vi "TrainEditor.vi"(8 "error in (no error)":errorcluster) -> (0 "error out":errorcluster, 1 "Clear Path":bool, 2 "PathData.Path":T1[](array[typedef]))   [LabVIEW 2014]
uses:
  Libraries/Contact Data/Contact.ctl
  Libraries/Contact Data/Position.ctl
  Libraries/Contact Data/Controls.ctl
  Libraries/Contact Data/DestinationCluster.ctl
  Libraries/Contact Data/DesinationControls.ctl
  Libraries/Contact Data/PathData.ctl
  PathFinder/Controls/ShortestPath.ctl
  Libraries/Contact Data/Command.ctl
  Libraries/Contact Data/Contact Data.lvlib
panel:
  in  "Clear Path":bool
  in  "Display Path":bool
  out "PathData":T2
  out "Speed":dbl
  out "SetSpeed":dbl
  out "Contact 2":T3
  in  "Use Copy?":bool
  in  "Destination Template":T6[](array[typedef])
  in  "Name":string
  out "Contact":T3
  in  "Update":i32=1000
  in  "Name display":T8(array[cluster])
  in  "Save ALL Single":bool
  in  "Save for all Dest only":bool
  in  "Destination Array":T6[](array[typedef])
  in  "Delete All":bool
  in  "Delete Index":bool
  in  "Save Destination only":bool
  in  "Load":bool
  out "Contacts":T3[](array[typedef])
  # "ID"
  # "UUID"
  # "Name"
  # "Select"
  # "Destination"
  # "Control"
  # "Timer"
  # "Set Time"
  # "TimeStamp"
  # "Repeat?"
  # "Optional Data"
  # "Distance"
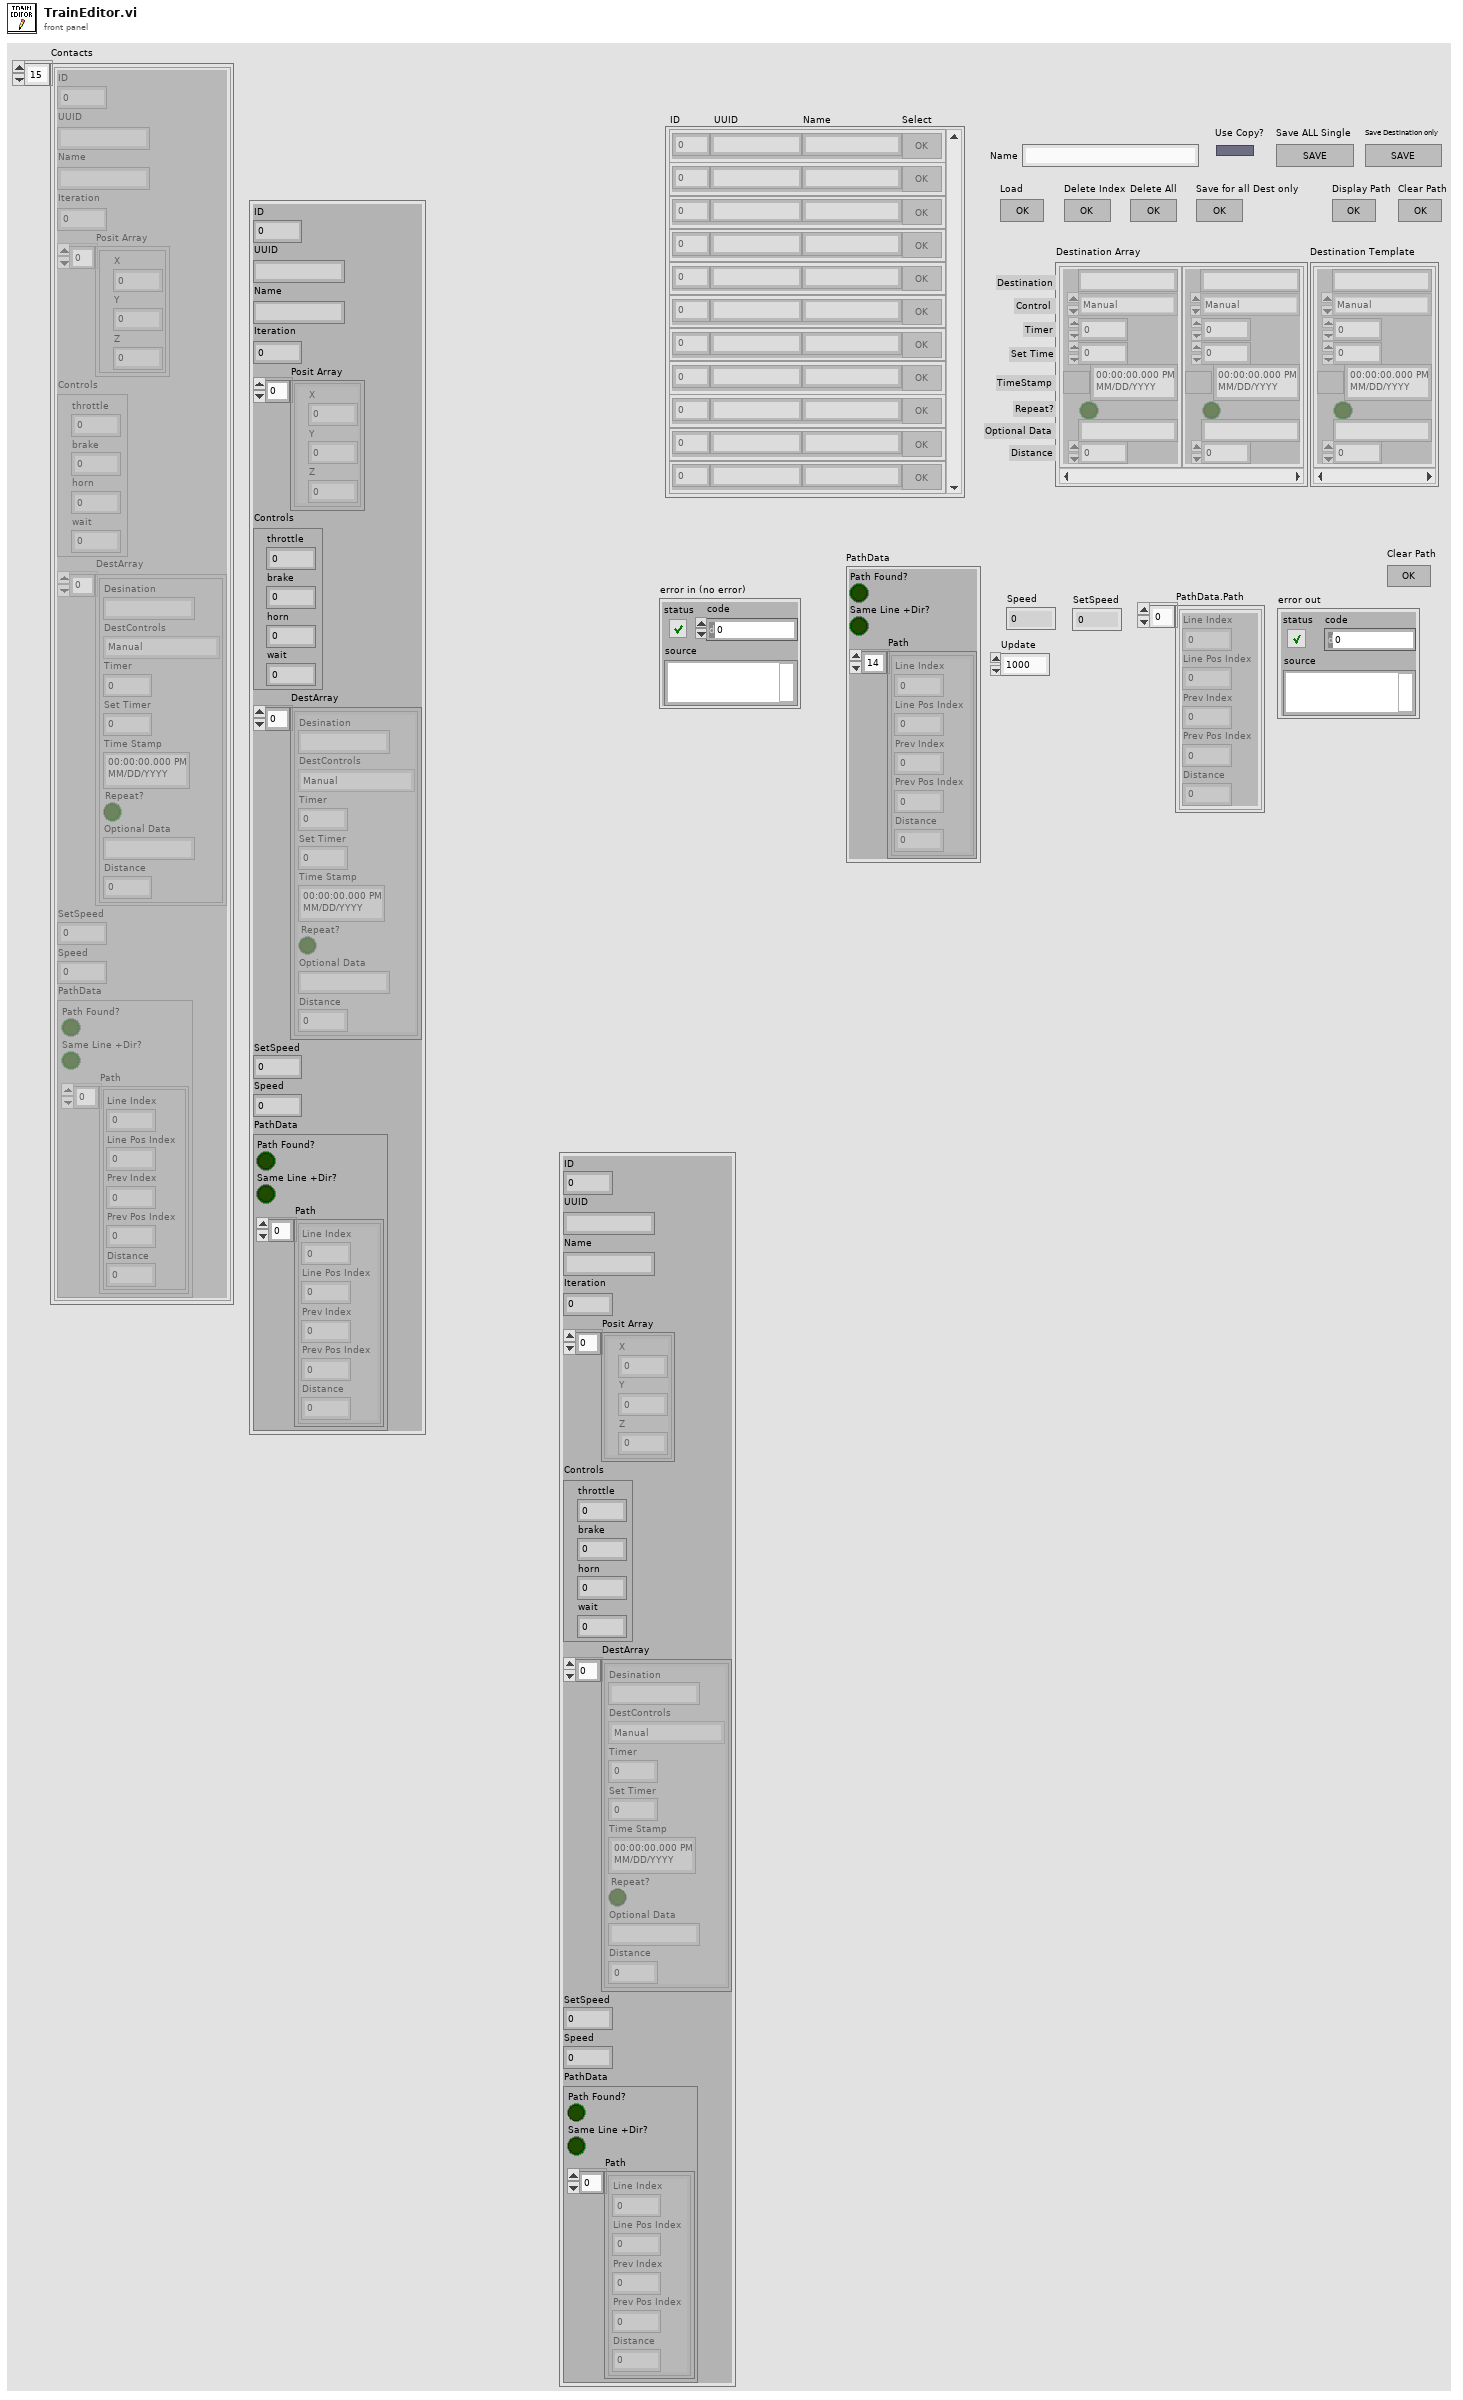
[diagram p1: front panel]
types:
  T1 = typedef "ShortestPath.ctl" = cluster{"Line Index":i32, "Line Pos Index ":i32, "Prev Index ":i32, "Prev Pos Index":i32, "Distance":dbl}
  T2 = typedef "Contact Data.lvlib/PathData.ctl" = cluster{"Path Found?":bool, "Same Line +Dir?":bool, "Path":T1[]}
  T3 = typedef "Contact Data.lvlib/Contact.ctl" = cluster{"ID":u32, "UUID":string, "Name":string, "Iteration":i32, "Posit Array":T4[], "Controls":T5, "DestArray":T6[], "SetSpeed":dbl, "Speed":dbl, "PathData":T2}
  T4 = typedef "Contact Data.lvlib/Position.ctl" = cluster{"X":dbl, "Y":dbl, "Z":dbl}
  T5 = typedef "Contact Data.lvlib/Controls.ctl" = cluster{"throttle":dbl, "brake":dbl, "horn":dbl, "wait":dbl}
  T6 = typedef "Contact Data.lvlib/DestinationCluster.ctl" = cluster{"Desination":string, "DestControls":T7, "Timer":u32, "Set Timer":u32, "Time Stamp":timestamp, "Repeat?":bool, "Optional Data":string, "Distance":dbl}
  T7 = typedef "Contact Data.lvlib/DesinationControls.ctl" = enum16{"Tracker", "Manual", "Stop", "Station DateTime", "Station Timer", "Maintain"}
  T8 = cluster{"ID":u32, "UUID":string, "Name":string, "Select":bool}[]
  T9 = enum32{"Invalid", "Standard", "Closed", "Hidden", "Minimized", "Maximized"}
  T10 = cluster{"ID":u32, "UUID":string, "Name":string, "Select":bool}
  T11 = typedef "Contact Data.lvlib/Command.ctl" = enum16{"Set All Contacts", "Load", "Save", "Get All Data", "Get Single Data (ID)", "Get Single Data", "Set Position", "Set Single Path", "Set Destinations", "Set Controls", "Remove Single Data", "Remove UUID Contact", "Set Single ALL", "Is Data Modified", "Import Data"}
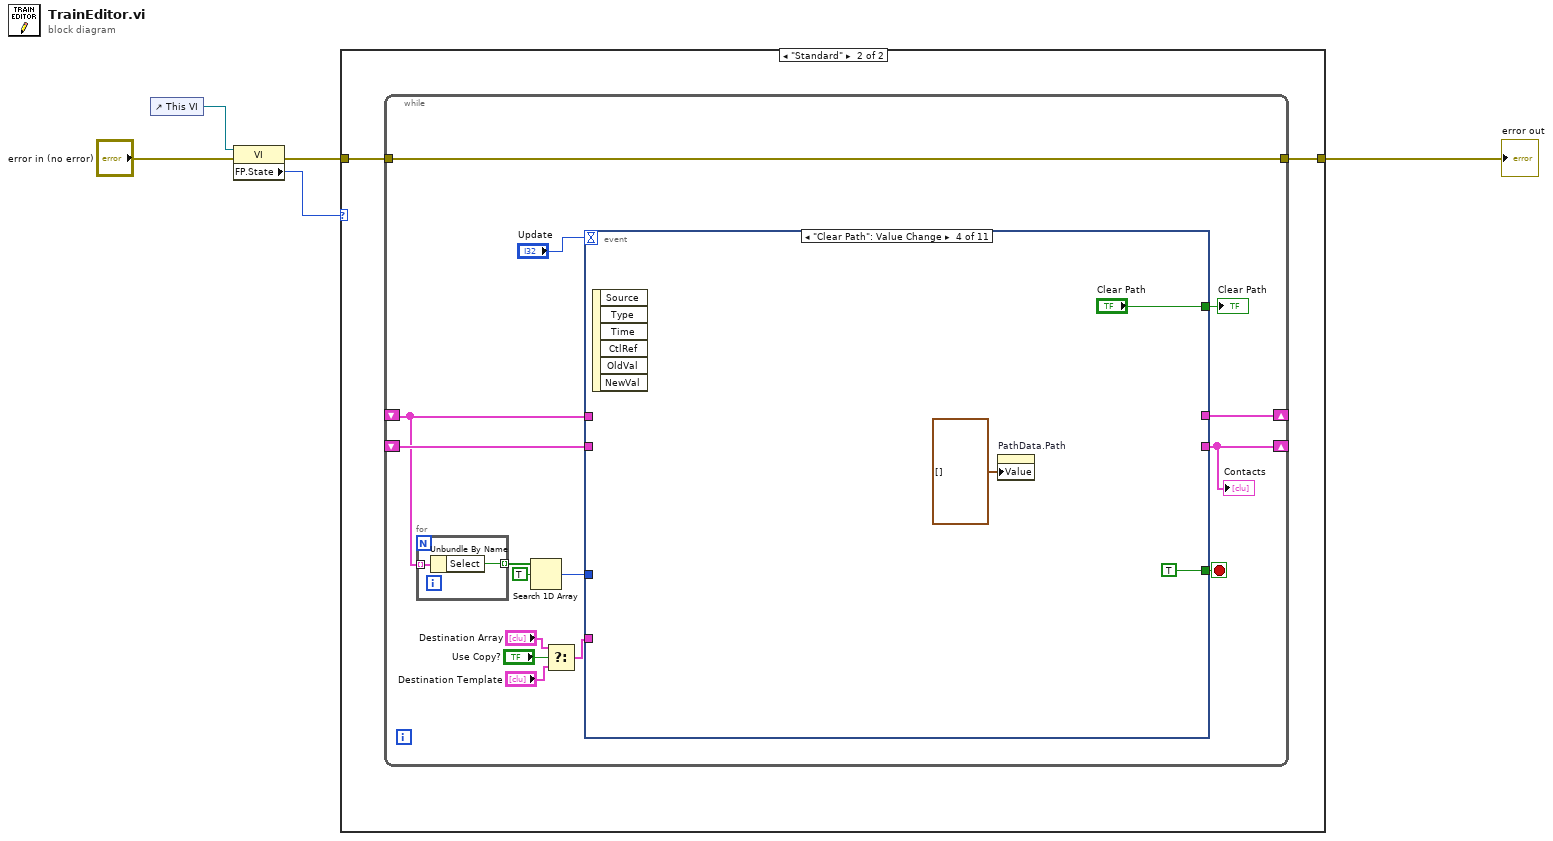
[diagram p0: block diagram]
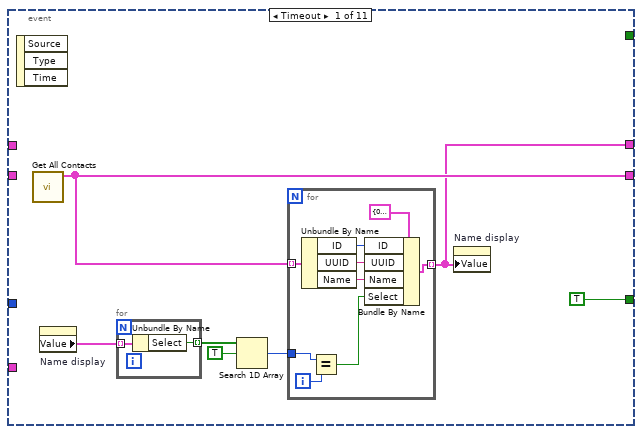
[diagram p3: hidden frame]
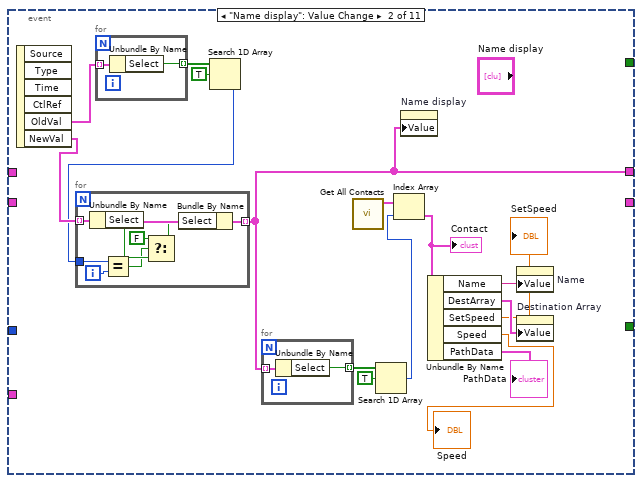
[diagram p4: hidden frame]
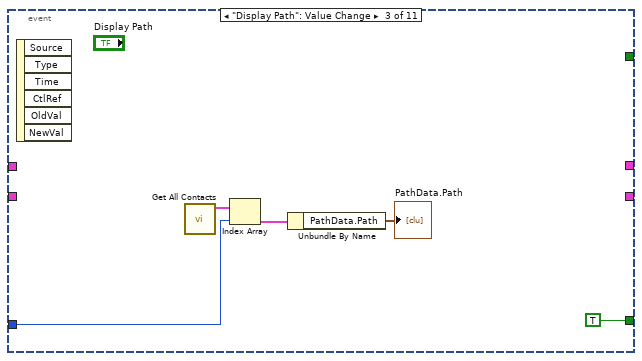
[diagram p5: hidden frame]
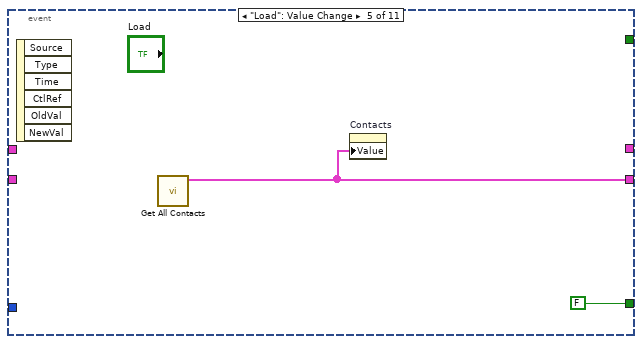
[diagram p6: hidden frame]
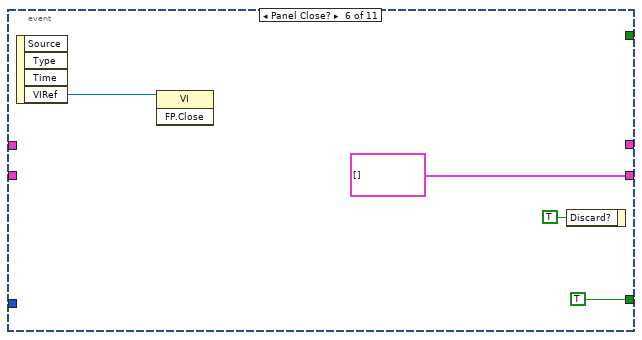
[diagram p7: hidden frame]
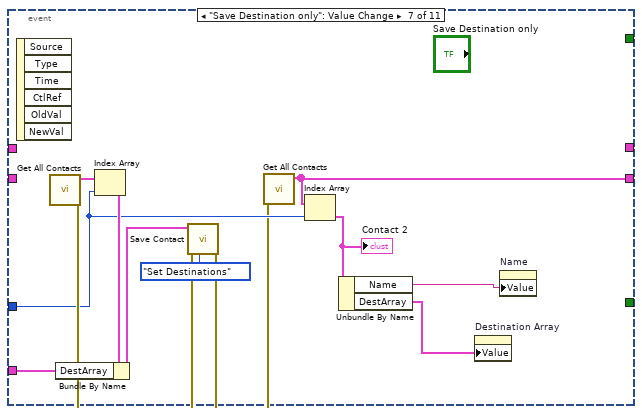
[diagram p8: hidden frame]
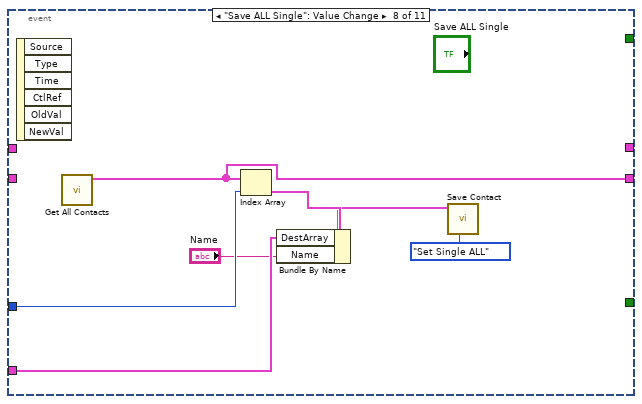
[diagram p9: hidden frame]
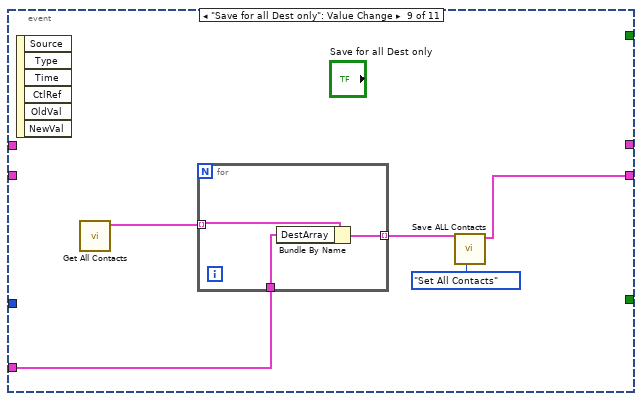
[diagram p10: hidden frame]
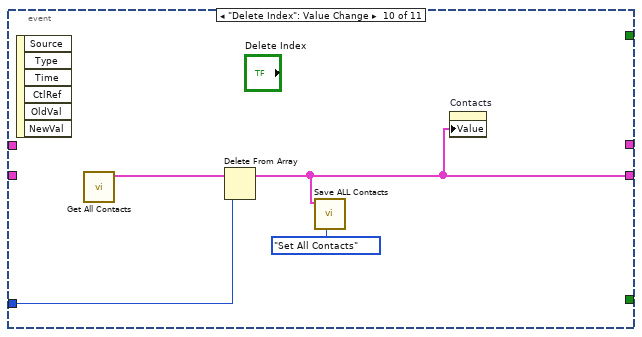
[diagram p11: hidden frame]
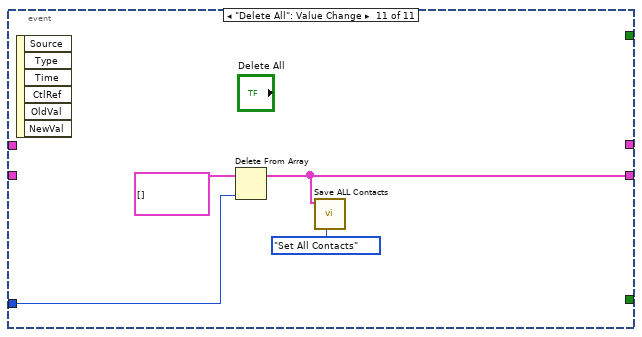
[diagram p12: hidden frame]
diagram:
  n1 = control-ref of="This VI"() -> (w5:refnum<vi>)
  n2 = property class="VI"(reference=w5, error in="error in (no error)") -> (error out=w1:errorcluster, "FP.State"=w4:T9)  [unwired: 1 out]
  n3 = case shown="\"Standard\"" w4 {
    tunnel: [w6 w7] -> w3
    tunnel: w1 -> [w6 w8]
    frame "Invalid", Default {
    }
    frame "Standard" {
      n4 = while {
        shift-right: [w11] -> _
        shift-left: _ -> [w21]
        shift-right: [w20] -> _
        shift-left: _ -> [w17]
        tunnel: w8 -> [w10]
        tunnel: [w10] -> w7
        stop <- w23 stop-if-true
        n5 = for {
          tunnel: w17 -> [w25] mode=indexing
          tunnel: [w24] -> w19 mode=indexing
          n6 = Unbundle By Name(w25) -> ("Select"=w24:bool)
        }
        n7 = Search 1D Array(1D array=w19, element=TRUE) -> (index of element=w16:i32)  [unwired: 1 in]
        n8 = Select(t="Destination Array", s="Use Copy?", f="Destination Template") -> (s? t:f=w13:T6[])
        n9 = event shown="[3] \"Clear Path\": Value Change" {
          selector: _ -> [_ _ _ _ _ _ _ _ _ _ _]
          dyn-events: _ -> [_ _ _ _ _ _ _ _ _ _ _]
          timeout: "Update" -> [_ _ _ _ _ _ _ _ _ _ _]
          tunnel: [TRUE _ TRUE TRUE FALSE TRUE _ _ _ _ _] -> w23
          tunnel: [w31 _ _ _ w80 T3[] [] ("Contacts") w88 w98 w106 w114 w118] -> w11
          tunnel: w21 -> [_ _ _ _ _ _ _ _ _ _ _]
          tunnel: w16 -> [_ _ w75 _ _ _ w90 w103 _ w116 w120]
          tunnel: w13 -> [_ _ _ _ _ _ w94 w100 w109 _ _]
          tunnel: [w26 w47 _ _ _ _ _ _ _ _ _] -> w20
          tunnel: w17 -> [_ _ _ _ _ _ _ _ _ _ _]
          tunnel: [_ _ _ "Clear Path" _ _ _ _ _ _ _] -> w9
          event Timeout {
            n10 = event-data() -> ()  [unwired: 1 in, 3 out]
            n11 = call "Get All Contacts.vi"() -> ("Contacts"=w31:T3[])  [unwired: 10 in, 1 out]
            n12 = property on="Name display" class="Arr (strict)"() -> ("Value"=w30:T8)  [unwired: 2 in, 2 out]
            n13 = for {
              tunnel: w30 -> [w34] mode=indexing
              tunnel: [w33] -> w29 mode=indexing
              n14 = Unbundle By Name(w34) -> ("Select"=w33:bool)
            }
            n15 = Search 1D Array(1D array=w29, element=TRUE) -> (index of element=w27:i32)  [unwired: 1 in]
            n16 = for {
              tunnel: w31 -> [w43] mode=indexing
              tunnel: [w35] -> w26 mode=indexing
              tunnel: w27 -> [w38]
              i -> [w37]
              n17 = Unbundle By Name(w43) -> ("ID"=w42:u32, "UUID"=w41:string, "Name"=w40:string)
              n18 = Equal?(x=w38, y=w37) -> (x = y?=w36:bool)
              n19 = Bundle By Name(cluster=T10 {"ID"=0, "UUID"="", "Name"="", "Select"=FALSE} ("Cluster"), "ID"=w42, "UUID"=w41, "Name"=w40, "Select"=w36) -> (w35:T10)
            }
            n20 = property on="Name display" class="Arr (strict)"("Value"=w26) -> ()  [unwired: 2 in, 2 out]
          }
          event "Name display": Value Change {
            n21 = event-data() -> ("OldVal"=w54:T8, "NewVal"=w52:T8)  [unwired: 1 in, 4 out]
            n22 = for {
              tunnel: w54 -> [w71] mode=indexing
              tunnel: [w70] -> w53 mode=indexing
              n23 = Unbundle By Name(w71) -> ("Select"=w70:bool)
            }
            n24 = Search 1D Array(1D array=w53, element=TRUE) -> (index of element=w51:i32)  [unwired: 1 in]
            n25 = for {
              tunnel: w52 -> [w69] mode=indexing
              tunnel: [w68] -> w47 mode=indexing
              tunnel: w51 -> [w62]
              i -> [w63]
              n26 = Unbundle By Name(w69) -> ("Select"=w67:bool)
              n27 = Equal?(x=w62, y=w63) -> (x = y?=w64:bool)
              n28 = Select(t=FALSE, s=w64, f=w67) -> (s? t:f=w65:bool)
              n29 = Bundle By Name(cluster=w69, "Select"=w65) -> (w68:T10)
            }
            n30 = for {
              tunnel: w47 -> [w61] mode=indexing
              tunnel: [w60] -> w50 mode=indexing
              n31 = Unbundle By Name(w61) -> ("Select"=w60:bool)
            }
            n32 = call "Get All Contacts.vi"() -> ("Contacts"=w58:T3[])  [unwired: 10 in, 1 out]
            n33 = Search 1D Array(1D array=w50, element=TRUE) -> (index of element=w48:i32)  [unwired: 1 in]
            n34 = Index Array(array=w58, index=w48) -> (element=w57:T3)
            "Contact" <- w57
            n35 = property on="Name display" class="Arr (strict)"("Value"=w47) -> ()  [unwired: 2 in, 2 out]
            n36 = Unbundle By Name(w57) -> ("Name"=w56:string, "DestArray"=w55:T6[], "SetSpeed"=→"SetSpeed":dbl, "Speed"=→"Speed":dbl, "PathData"=→"PathData":T2)
            n37 = property on="Name" class="Str"("Value"=w56) -> ()  [unwired: 2 in, 2 out]
            n38 = property on="Destination Array" class="Arr (strict)"("Value"=w55) -> ()  [unwired: 2 in, 2 out]
          }
          event "Display Path": Value Change {
            n39 = event-data() -> ()  [unwired: 1 in, 6 out]
            n40 = call "Get All Contacts.vi"() -> ("Contacts"=w76:T3[])  [unwired: 10 in, 1 out]
            n41 = Index Array(array=w76, index=w75) -> (element=w74:T3)
            n42 = Unbundle By Name(w74) -> ("PathData.Path"=→"PathData.Path":T1[])
          }
          event "Clear Path": Value Change {
            n43 = event-data() -> ()  [unwired: 1 in, 6 out]
            n44 = property on="PathData.Path" class="Arr (strict)"("Value"=T1[] [] ("PathData.Path")) -> ()  [unwired: 2 in, 2 out]
          }
          event "Load": Value Change {
            n45 = event-data() -> ()  [unwired: 1 in, 6 out]
            n46 = call "Get All Contacts.vi"() -> ("Contacts"=w80:T3[])  [unwired: 10 in, 1 out]
            n47 = property on="Contacts" class="Arr (strict)"("Value"=w80) -> ()  [unwired: 2 in, 2 out]
          }
          event Panel Close? {
            n48 = event-data() -> ("VIRef"=w82:refnum<vi>)  [unwired: 1 in, 3 out]
            n49 = invoke class="VI" method="FP.Close"(reference=w82) -> ()  [unwired: 2 in, 3 out]
            n50 = event-data("Discard?"=TRUE) -> ()  [unwired: 1 in, 1 out]
          }
          event "Save Destination only": Value Change {
            n51 = event-data() -> ()  [unwired: 1 in, 6 out]
            n52 = call "Get All Contacts.vi"() -> ("error out"=w92:errorcluster, "Contacts"=w93:T3[])  [unwired: 10 in]
            n53 = Index Array(array=w93, index=w90) -> (element=w96:T3)
            n54 = Bundle By Name(cluster=w96, "DestArray"=w94) -> (w95:T3)
            n55 = call "Save Contact.vi"("Command"=Command."Set Destinations", "error in (no error)"=w92, "Contact"=w95) -> ("error out"=w89:errorcluster)  [unwired: 7 in, 1 out]
            n56 = call "Get All Contacts.vi"("error in (no error)"=w89) -> ("Contacts"=w88:T3[])  [unwired: 9 in, 1 out]
            n57 = Index Array(array=w88, index=w90) -> (element=w91:T3)
            "Contact 2" <- w91
            n58 = Unbundle By Name(w91) -> ("Name"=w87:string, "DestArray"=w86:T6[])
            n59 = property on="Destination Array" class="Arr (strict)"("Value"=w86) -> ()  [unwired: 2 in, 2 out]
            n60 = property on="Name" class="Str"("Value"=w87) -> ()  [unwired: 2 in, 2 out]
          }
          event "Save ALL Single": Value Change {
            n61 = event-data() -> ()  [unwired: 1 in, 6 out]
            n62 = call "Get All Contacts.vi"() -> ("Contacts"=w98:T3[])  [unwired: 10 in, 1 out]
            n63 = Index Array(array=w98, index=w103) -> (element=w102:T3)
            n64 = Bundle By Name(cluster=w102, "DestArray"=w100, "Name"="Name") -> (w101:T3)
            n65 = call "Save Contact.vi"("Command"=Command."Set Single ALL", "Contact"=w101) -> ()  [unwired: 8 in, 2 out]
          }
          event "Save for all Dest only": Value Change {
            n66 = event-data() -> ()  [unwired: 1 in, 6 out]
            n67 = call "Get All Contacts.vi"() -> ("Contacts"=w105:T3[])  [unwired: 10 in, 1 out]
            n68 = for {
              tunnel: w109 -> [w112]
              tunnel: w105 -> [w111] mode=indexing
              tunnel: [w110] -> w107 mode=indexing
              n69 = Bundle By Name(cluster=w111, "DestArray"=w112) -> (w110:T3)
            }
            n70 = call "Save ALL Contacts.vi"("Command"=Command."Set All Contacts", "Contact in"=w107) -> ("Contact out"=w106:T3[])  [unwired: 8 in, 1 out]
          }
          event "Delete Index": Value Change {
            n71 = event-data() -> ()  [unwired: 1 in, 6 out]
            n72 = call "Get All Contacts.vi"() -> ("Contacts"=w113:T3[])  [unwired: 10 in, 1 out]
            n73 = Delete From Array(array=w113, index=w116) -> (array with subset deleted=w114:T3[])  [unwired: 1 in, 1 out]
            n74 = call "Save ALL Contacts.vi"("Command"=Command."Set All Contacts", "Contact in"=w114) -> ()  [unwired: 8 in, 2 out]
            n75 = property on="Contacts" class="Arr (strict)"("Value"=w114) -> ()  [unwired: 2 in, 2 out]
          }
          event "Delete All": Value Change {
            n76 = event-data() -> ()  [unwired: 1 in, 6 out]
            n77 = Delete From Array(array=T3[] [], index=w120) -> (array with subset deleted=w118:T3[])  [unwired: 1 in, 1 out]
            n78 = call "Save ALL Contacts.vi"("Command"=Command."Set All Contacts", "Contact in"=w118) -> ()  [unwired: 8 in, 2 out]
          }
        }
        "Contacts" <- w11
        "Clear Path" <- w9
      }
    }
  }
  "error out" <- w3
